vi "newsub2.vi"(11 "x":dbl) -> (3 "Numeric":dbl)   [LabVIEW 2015]
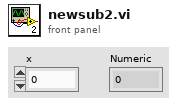
[diagram p1: front panel]
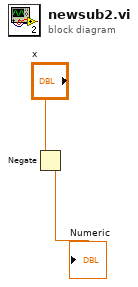
[diagram p0: block diagram]
diagram:
  n1 = Negate(x="x") -> (-x=→"Numeric":dbl)
